vi "json_encode.vi"(8 "error in (no error)":errorcluster, 10 "key":string, 11 "variant":variant) -> (0 "error out":errorcluster, 3 "json":string)   [LabVIEW 2017, in "rethinkdb.lvlib"]
uses:
  rethinkdb.lvlib
  <vilib>/Utility/Data Type/NI_Data Type.lvlib
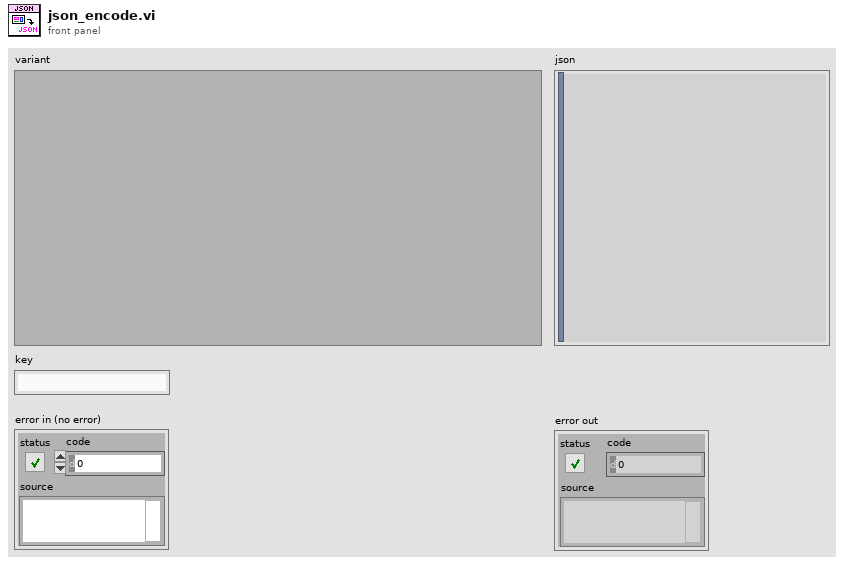
[diagram p1: front panel]
types:
  T1 = typedef "NI_Data Type.lvlib/Data Type.ctl" = enum8{"Invalid Type", "Void", "I8", "I16", "I32", "I64", "U8", "U16", "U32", "U64", "Single Float", "Double Float", "Extended Float", "Single Complex", "Double Complex", "Extended Complex", "Enum U8", "Enum U16", "Enum U32", "Enum U64", "Single Float With Unit", "Double Float With Unit", "Extended Float With Unit", "Single Complex with Unit", "Double Complex with Unit", "Extended Complex with Unit", "Boolean", "String", "Path", "Picture", "Tag", "Array", "Cluster", "Variant", "LV Variant", "Waveform", "Timestamp", "Digital Waveform", "Digital Data", "ExpressData", "Refnum", "External Data", "VI", "Poly VI", "LabVIEW Class Instance", "Fixed Point"}
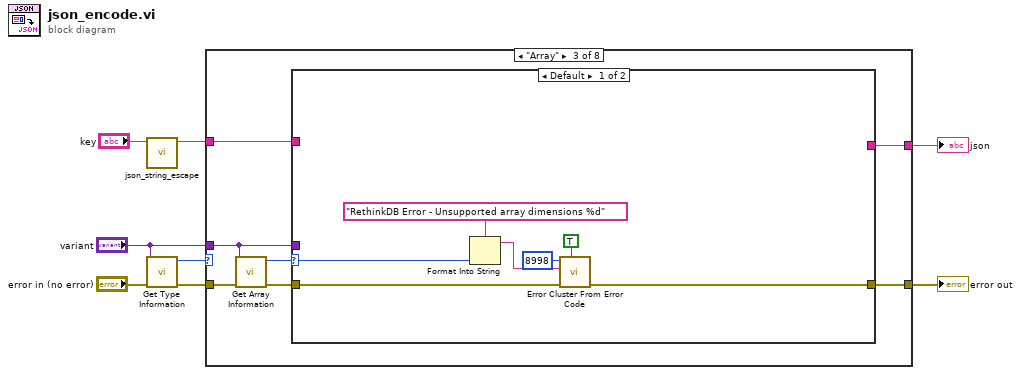
[diagram p0: block diagram]
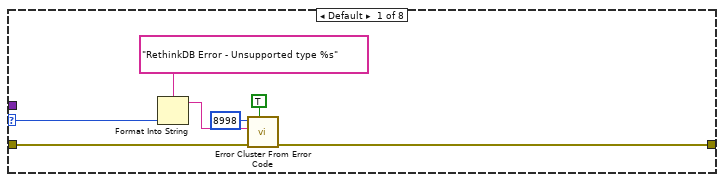
[diagram p2: hidden frame]
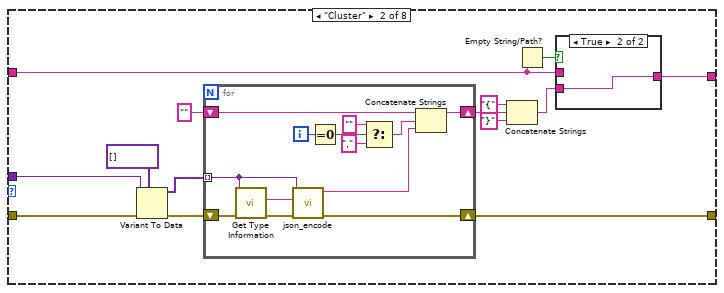
[diagram p3: hidden frame]
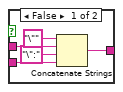
[diagram p4: hidden frame]
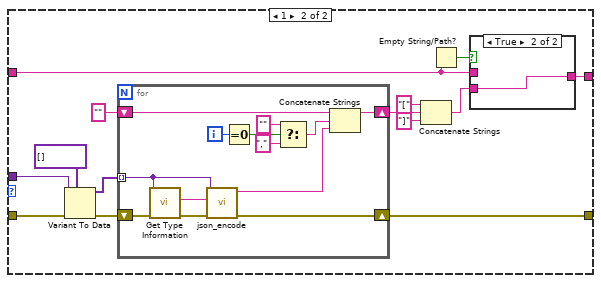
[diagram p5: hidden frame]
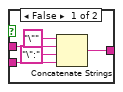
[diagram p6: hidden frame]
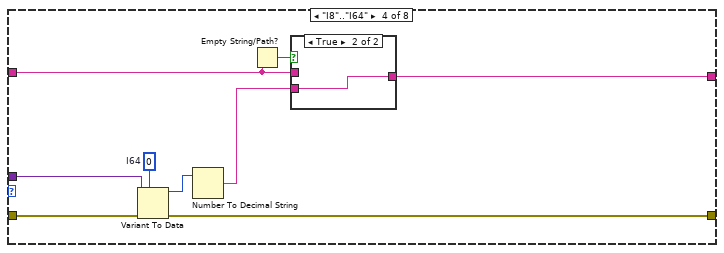
[diagram p7: hidden frame]
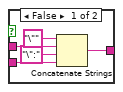
[diagram p8: hidden frame]
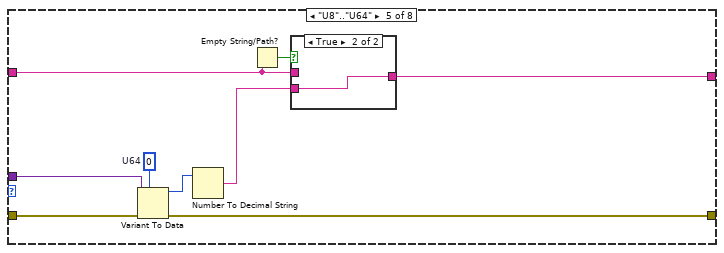
[diagram p9: hidden frame]
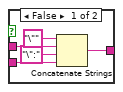
[diagram p10: hidden frame]
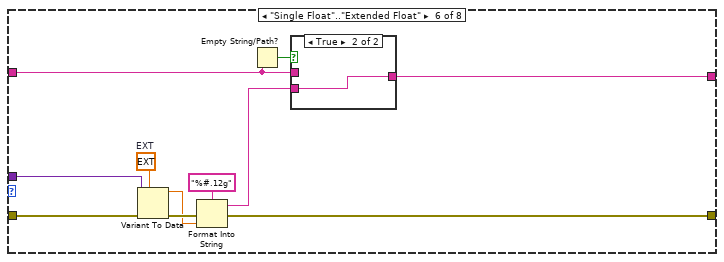
[diagram p11: hidden frame]
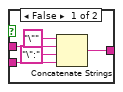
[diagram p12: hidden frame]
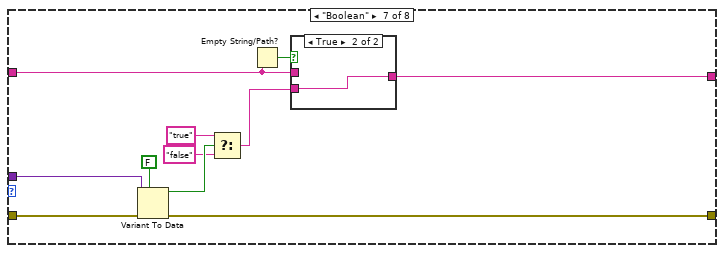
[diagram p13: hidden frame]
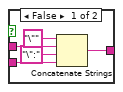
[diagram p14: hidden frame]
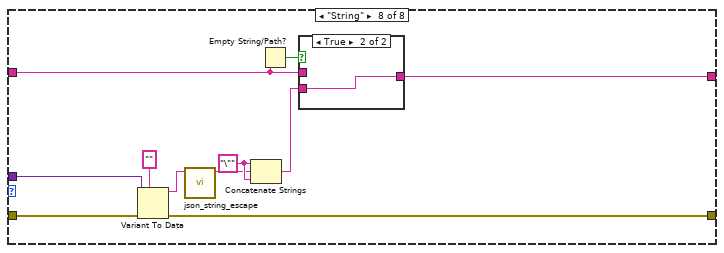
[diagram p15: hidden frame]
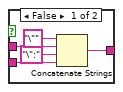
[diagram p16: hidden frame]
diagram:
  n1 = call "json_string_escape.vi"("string"="key") -> ("escaped string"=w1:string)  [unwired: 10 in]
  n2 = call <vilib>:"Get Type Information.vi"("error in (no error)"="error in (no error)", "Variant"="variant") -> ("error out"=w5:errorcluster, "Type"=w7:T1)  [unwired: 5 in, 3 out]
  n3 = case shown="\"Array\"" w7 {
    selector: w7 -> [w11 _ _ _ _ _ _ _]
    tunnel: "variant" -> [_ w28 w51 w103 w118 w135 w152 w169]
    tunnel: w5 -> [w15 w29 w52 w104 w119 w136 w153 w170]
    tunnel: [w14 w26 w55 w99 w114 w129 w147 w165] -> w4
    tunnel: [_ w21 w54 w98 w113 w132 w151 w168] -> w3
    tunnel: w1 -> [_ w20 w53 w97 w112 w131 w150 w167]
    frame Default {
      n4 = Format Into String(format string="RethinkDB Error - Unsupported type %s" ("error message (\"\")"), w11) -> (resulting string=w9:string)  [unwired: 2 in, 1 out]
      n5 = call <vilib>:"Error Cluster From Error Code.vi"("show call chain? (False)"=TRUE, "error in (no error)"=w15, "error message (\"\")"=w9, "error code (0)"=8998) -> ("error out"=w14:errorcluster)  [unwired: 5 in]
    }
    frame "Cluster" {
      n6 = Variant To Data(error in=w29, type=variant[] [], Variant=w28) -> (data=w24:variant[], error out=w25:errorcluster)
      n7 = for {
        shift-right: [w48] -> w26
        shift-left: w25 -> [w47]
        tunnel: w24 -> [w45] mode=indexing
        shift-right: [w42] -> w19
        shift-left: "" -> [w43]
        i -> [w41]
        n8 = call <vilib>:"Get Type Information.vi"("error in (no error)"=w47, "Variant"=w45) -> ("error out"=w46:errorcluster, "Name"=w44:string)  [unwired: 5 in, 3 out]
        n9 = call "json_encode.vi"("error in (no error)"=w46, "key"=w44, "variant"=w45) -> ("error out"=w48:errorcluster, "json"=w40:string)  [unwired: 7 in]
        n10 = Equal To 0?(x=w41) -> (x = 0?=w39:bool)
        n11 = Select(t="", s=w39, f="," ("string")) -> (s? t:f=w36:string)
        n12 = Concatenate Strings(w43, w36, w40) -> (w42:string)
      }
      n13 = Concatenate Strings("{" ("string"), w19, "}" ("string")) -> (w18:string)
      n14 = Empty String/Path?(string/path=w20) -> (empty?=w22:bool)
      n15 = case shown="True" w22 {
        tunnel: w18 -> [w32 w35]
        tunnel: [w31 w35] -> w21
        tunnel: w20 -> [w30 _]
        frame False {
          n16 = Concatenate Strings("\"" ("string"), w30, "\":" ("string"), w32) -> (w31:string)
        }
        frame True {
        }
      }
    }
    frame "Array" {
      n17 = call <vilib>:"Get Array Information.vi"("error in (no error)"=w52, "Variant"=w51) -> ("error out"=w50:errorcluster, "Number of Dimensions"=w49:i32)  [unwired: 6 in, 2 out]
      n18 = case shown="Default" w49 {
        selector: w49 -> [w57 _]
        tunnel: [w56 w75] -> w55
        tunnel: [_ w70] -> w54
        tunnel: w53 -> [_ w69]
        tunnel: w51 -> [_ w64]
        tunnel: w50 -> [w58 w63]
        frame Default {
          n19 = Format Into String(format string="RethinkDB Error - Unsupported array dimensions %d" ("error message (\"\")"), w57) -> (resulting string=w59:string)  [unwired: 2 in, 1 out]
          n20 = call <vilib>:"Error Cluster From Error Code.vi"("show call chain? (False)"=TRUE, "error in (no error)"=w58, "error message (\"\")"=w59, "error code (0)"=8998) -> ("error out"=w56:errorcluster)  [unwired: 5 in]
        }
        frame 1 {
          n21 = Variant To Data(error in=w63, type=variant[] [], Variant=w64) -> (data=w73:variant[], error out=w74:errorcluster)
          n22 = for {
            shift-right: [w95] -> w75
            shift-left: w74 -> [w94]
            tunnel: w73 -> [w92] mode=indexing
            shift-right: [w89] -> w68
            shift-left: "" -> [w90]
            i -> [w88]
            n23 = call <vilib>:"Get Type Information.vi"("error in (no error)"=w94, "Variant"=w92) -> ("error out"=w93:errorcluster, "Name"=w91:string)  [unwired: 5 in, 3 out]
            n24 = call "json_encode.vi"("error in (no error)"=w93, "key"=w91, "variant"=w92) -> ("error out"=w95:errorcluster, "json"=w87:string)  [unwired: 7 in]
            n25 = Equal To 0?(x=w88) -> (x = 0?=w86:bool)
            n26 = Select(t="", s=w86, f="," ("string")) -> (s? t:f=w83:string)
            n27 = Concatenate Strings(w90, w83, w87) -> (w89:string)
          }
          n28 = Concatenate Strings("[" ("string"), w68, "]" ("string")) -> (w67:string)
          n29 = Empty String/Path?(string/path=w69) -> (empty?=w71:bool)
          n30 = case shown="True" w71 {
            tunnel: w67 -> [w79 w82]
            tunnel: [w78 w82] -> w70
            tunnel: w69 -> [w77 _]
            frame False {
              n31 = Concatenate Strings("\"" ("string"), w77, "\":" ("string"), w79) -> (w78:string)
            }
            frame True {
            }
          }
        }
      }
    }
    frame "I8".."I64" {
      w102 = i64 0  # I64
      n32 = Variant To Data(error in=w104, type=w102, Variant=w103) -> (data=w101:i64, error out=w99:errorcluster)
      n33 = Number To Decimal String(number=w101) -> (decimal integer string=w100:string)  [unwired: 1 in]
      n34 = Empty String/Path?(string/path=w97) -> (empty?=w96:bool)
      n35 = case shown="True" w96 {
        tunnel: w100 -> [w107 w110]
        tunnel: [w106 w110] -> w98
        tunnel: w97 -> [w105 _]
        frame False {
          n36 = Concatenate Strings("\"" ("string"), w105, "\":" ("string"), w107) -> (w106:string)
        }
        frame True {
        }
      }
    }
    frame "U8".."U64" {
      w117 = u64 0  # U64
      n37 = Variant To Data(error in=w119, type=w117, Variant=w118) -> (data=w116:u64, error out=w114:errorcluster)
      n38 = Number To Decimal String(number=w116) -> (decimal integer string=w115:string)  [unwired: 1 in]
      n39 = Empty String/Path?(string/path=w112) -> (empty?=w111:bool)
      n40 = case shown="True" w111 {
        tunnel: w115 -> [w122 w125]
        tunnel: [w121 w125] -> w113
        tunnel: w112 -> [w120 _]
        frame False {
          n41 = Concatenate Strings("\"" ("string"), w120, "\":" ("string"), w122) -> (w121:string)
        }
        frame True {
        }
      }
    }
    frame "Single Float".."Extended Float" {
      w134 = ext 0.0  # EXT
      n42 = Variant To Data(error in=w136, type=w134, Variant=w135) -> (data=w128:ext, error out=w133:errorcluster)
      n43 = Format Into String(format string="%#.12g", error in=w133, w128) -> (resulting string=w126:string, error out=w129:errorcluster)  [unwired: 1 in]
      n44 = Empty String/Path?(string/path=w131) -> (empty?=w130:bool)
      n45 = case shown="True" w130 {
        tunnel: w126 -> [w139 w142]
        tunnel: [w138 w142] -> w132
        tunnel: w131 -> [w137 _]
        frame False {
          n46 = Concatenate Strings("\"" ("string"), w137, "\":" ("string"), w139) -> (w138:string)
        }
        frame True {
        }
      }
    }
    frame "Boolean" {
      n47 = Variant To Data(error in=w153, type=FALSE, Variant=w152) -> (data=w146:bool, error out=w147:errorcluster)
      n48 = Select(t="true", s=w146, f="false") -> (s? t:f=w145:string)
      n49 = Empty String/Path?(string/path=w150) -> (empty?=w149:bool)
      n50 = case shown="True" w149 {
        tunnel: w145 -> [w156 w159]
        tunnel: [w155 w159] -> w151
        tunnel: w150 -> [w154 _]
        frame False {
          n51 = Concatenate Strings("\"" ("string"), w154, "\":" ("string"), w156) -> (w155:string)
        }
        frame True {
        }
      }
    }
    frame "String" {
      w162 = "\"" ("string")
      n52 = Variant To Data(error in=w170, type="", Variant=w169) -> (data=w161:string, error out=w165:errorcluster)
      n53 = call "json_string_escape.vi"("string"=w161) -> ("escaped string"=w160:string)  [unwired: 10 in]
      n54 = Concatenate Strings(w162, w160, w162) -> (w163:string)
      n55 = Empty String/Path?(string/path=w167) -> (empty?=w166:bool)
      n56 = case shown="True" w166 {
        tunnel: w163 -> [w173 w176]
        tunnel: [w172 w176] -> w168
        tunnel: w167 -> [w171 _]
        frame False {
          n57 = Concatenate Strings("\"" ("string"), w171, "\":" ("string"), w173) -> (w172:string)
        }
        frame True {
        }
      }
    }
  }
  "json" <- w3
  "error out" <- w4
